vi "枚举所有的com口之后找到对应的字符串.vi"() -> ()   [LabVIEW 2018]
panel:
  out "数组 3":i32[](array[numeric])
  out "数组 2":u32[](array[numeric])
  out "匹配后偏移量":i32
  out "匹配子字符串":string
  out "数组":string[](array[string])
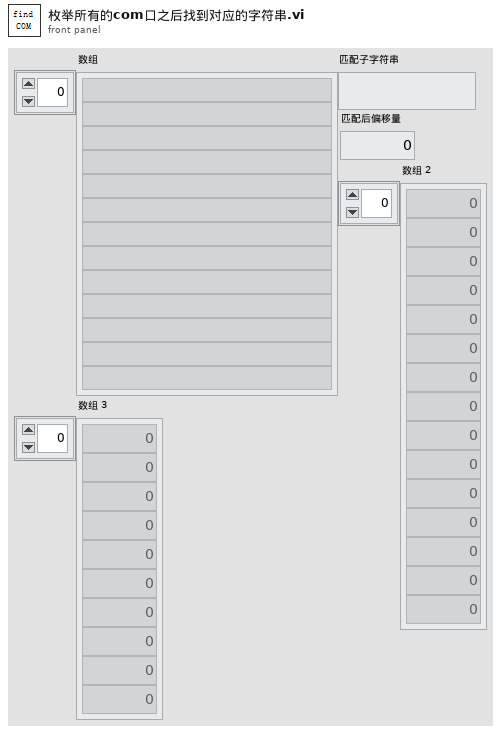
[diagram p1: front panel]
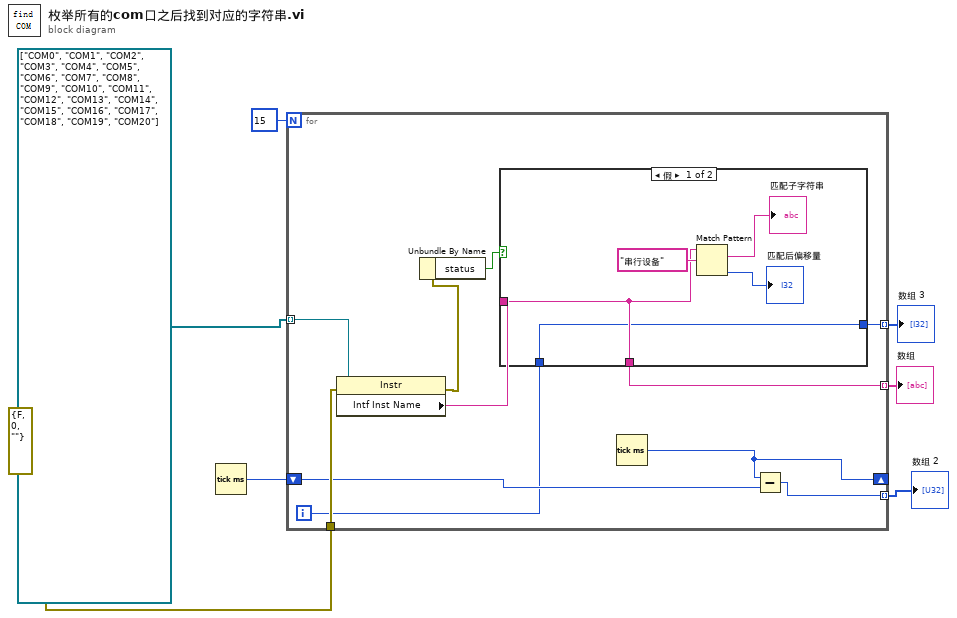
[diagram p0: block diagram]
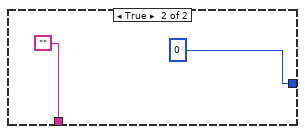
[diagram p2: hidden frame]
diagram:
  n1 = Tick Count (ms)() -> (millisecond timer value=w3:u32)
  n2 = for {
    N: 15 -> [_]
    tunnel: refnum<visa-resource-name>[] ["COM0", "COM1", "COM2", "COM3", "COM4", "COM5", "COM6", "COM7", "COM8", "COM9", "COM10", "COM11", "COM12", "COM13", "COM14", "COM15", "COM16", "COM17", "COM18", "COM19", "COM20"] ("添加的数组") -> [w18] mode=indexing
    tunnel: [w14] -> w6 mode=indexing
    tunnel: errorcluster {"status"=FALSE, "code"=0, "source"=""} ("error in (no error)") -> [w17]
    tunnel: [w10] -> w2 mode=indexing
    shift-right: [w8] -> _
    shift-left: w3 -> [w12]
    tunnel: [w9] -> w1 mode=indexing
    i -> [w11]
    n3 = property class="Instr"(reference=w18, error in=w17) -> (error out=w16:errorcluster, "Intf Inst Name"=w13:string)  [unwired: 1 out]
    n4 = Unbundle By Name(w16) -> ("status"=w15:bool)
    n5 = case shown="假" w15 {
      tunnel: [w22 ""] -> w14
      tunnel: w13 -> [w22 _]
      tunnel: w11 -> [w19 _]
      tunnel: [w19 0] -> w10
      frame False {
        n6 = Match Pattern(string=w22, regular expression="串行设备" ("正则表达式")) -> (match substring=→"匹配子字符串":string, offset past match=→"匹配后偏移量":i32)  [unwired: 1 in, 2 out]
      }
      frame True {
      }
    }
    n7 = Tick Count (ms)() -> (millisecond timer value=w8:u32)
    n8 = Subtract(x=w8, y=w12) -> (x-y=w9:u32)
  }
  "数组" <- w6
  "数组 2" <- w1
  "数组 3" <- w2
